vi "Delete Host Key Database Refnum.vi"(8 "error in (no error)":errorcluster, 11 "host key database":T1) -> (0 "error out":errorcluster, 3 "LIBSSH2_KNOWNHOSTS*":u64)   [LabVIEW 2013, in "libssh2.lvlib"]
uses:
  libssh2.lvlib
  Host Key Database Refnum.ctl
  Host Key Database Refnum Data.ctl
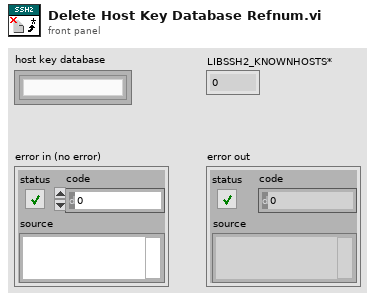
[diagram p1: front panel]
types:
  T1 = typedef "libssh2.lvlib/Host Key Database Refnum.ctl" = refnum<k1>
  T2 = typedef "libssh2.lvlib/Host Key Database Refnum Data.ctl" = cluster{"LIBSSH2_KNOWNHOSTS*":u64, "semaphore":T3}
  T3 = typedef "Semaphore RefNum" = refnum<k1>
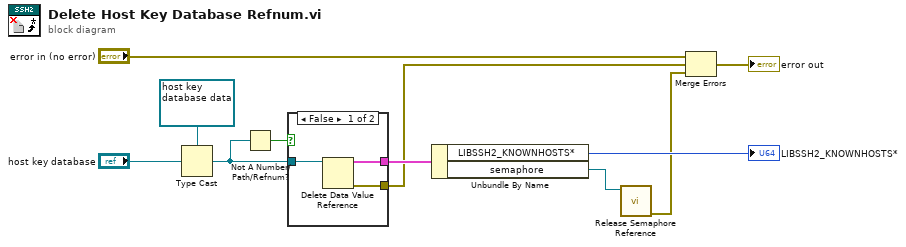
[diagram p0: block diagram]
diagram:
  n1 = Type Cast(type=refnum<data-value> refnum ("data value reference"), x="host key database") -> (*(type *) &x=w8:refnum<data-value>)
  n2 = Not A Number/Path/Refnum?(number/path/refnum=w8) -> (NaN/Path/Refnum?=w7:bool)
  n3 = case shown="False" w7 {
    tunnel: [w14 _] -> w10
    tunnel: [w13 _] -> w9
    tunnel: w8 -> [w12 _]
    frame False {
      n4 = Delete Data Value Reference(data value reference=w12) -> (data value=w14:T2, error out=w13:errorcluster)  [unwired: 1 in]
    }
    frame True {
    }
  }
  n5 = Unbundle By Name(w10) -> ("LIBSSH2_KNOWNHOSTS*"=→"LIBSSH2_KNOWNHOSTS*":u64, "semaphore"=w3:T3)
  n6 = call <vilib>:"Release Semaphore Reference.vi"("semaphore"=w3) -> ("error out"=w1:errorcluster)  [unwired: 9 in, 1 out]
  n7 = Merge Errors("error in (no error)", w9, w1) -> (→"error out":errorcluster)
